vi "Camera.vi"(0 "Camera in":refnum<class "Camera.lvclass">, 1 "Stop":bool, 3 "Cluster":T1={"Bayer"={"Algorithm"=0, "Gain R"=1.0, "Gain B"=1.0, "Gain G"=1.0, "Pattern"=5}, "Acquisition Control"={"Trigger Selector"=0, "Acquisition Frame Rate"=0.0, "Exposure Time"=0.0, "Acquisition Frame Rate Target"=0.0}, "Analog Control"={"Black Level"=1.5, "Gain Selector"=10, "Gain"=1.0}} {"Analog Control"."Gain" min=1.0 max=15.0; "Analog Control"."Gain Selector" items=["Analog All"=10, "Digital All"=20]; "Analog Control"."Black Level" min=0.0 max=255.9375; "Acquisition Control"."Acquisition Frame Rate Target" min=0.001 max=150000000.0; "Acquisition Control"."Exposure Time" min=27.793333333333333 max=1048539.7933333333; "Acquisition Control"."Acquisition Frame Rate" min=0.9536888685435264 max=30.757874015748033; "Acquisition Control"."Trigger Selector" items=["Frame Start"=3, "Exposure Start"=10]; "Bayer"."Pattern" items=["Use hardware value"=5, "None"=0, "GB"=1, "GR"=2, "BG"=3, "RG"=4]; "Bayer"."Gain G" min=0.0 max=3.999; "Bayer"."Gain B" min=0.0 max=3.999; "Bayer"."Gain R" min=0.0 max=3.999; "Bayer"."Algorithm" items=["Bilinear", "VNG"]}, 4 "BCG Image Processing":T6={"Brightness"=128.0, "Contrast"=45.0, "Gamma"=1.0} {"Brightness" scale=0.0..400.0; "Contrast" scale=0.0..90.0; "Gamma" scale=0.005..5.0}, 5 "error in (no error)":errorcluster, 6 "Machine Vision":T7, 7 "Camera settings":T5={"Gamma"=1.0, "Gain"=7, "Sharpness"=0, "Contrast"=0.009999999999999995, "Exposure"=0.0004073180282999787} {"Exposure" min=0.000244140625 max=0.5 scale=0.0002..0.5; "Contrast" min=0.0 max=1.0 scale=0.001..1.0; "Sharpness" min=0 max=2 step=1 scale=0.0..2.0; "Gain" min=0 max=100 step=1 scale=0.1..100.0; "Gamma" min=0.01 max=10.0 scale=0.01..10.0}, 12 "Loop 0":bool, 13 "Override presets":bool) -> (9 "All Matches XY":sgl[][](array[numeric]), 11 "Used Edges (Adv. Straight Edge 1)":cluster{"Edge Information":T2[]}[](array[cluster]) {"Edge Information"."Distance (Real-World)" format="%.2f"; "Edge Information"."Location (Real-World)"."Y" format="%.2g"; "Edge Information"."Location (Real-World)"."X" format="%.2f"; "Edge Information"."Noise" format="%.2f"; "Edge Information"."Location (Pixel)"."Y" format="%.2g"; "Edge Information"."Location (Pixel)"."X" format="%.2f"; "Edge Information"."Strength" format="%.2f"; "Edge Information"."Distance (Pixel)" format="%.2f"}, 14 "Camera out":refnum<class "Camera.lvclass">, 15 "output cluster":T4, 16 "pattern matching":T3 {"Correlation Score" format="%.2f"; "Target Template Curve Score" format="%.2f"; "Template Target Curve Score" format="%.2f"; "Bounding Box"."y" format="%.2f"; "Bounding Box"."x" format="%.2f"; "Position"."y" format="%.2f"; "Position"."x" format="%.2f"; "Score" format="%.2f"; "Scale" format="%.2f"; "Angle" format="%.2f"; "Occlusion %" format="%.2f"}, 17 "Image":T8(plugin-control), 18 "Camera":dbl[](array[numeric]), 19 "error out":errorcluster)   [LabVIEW 2021, in "Camera.lvclass"]
uses:
  Camera.lvclass
  Machine Vision.ctl
  Image processing.ctl
  Camera settings.ctl
  <vilib>/vision/Pattern Matching.llb/IMAQ GM Match Report.ctl
  <vilib>/vision/Measure.llb/Edge New.ctl
  <vilib>/Analysis/baseanly.llb/Mean (DBL).vi
  <vilib>/Utility/file.llb/Read Delimited Spreadsheet (string).vi
  <vilib>/vision/NI_Vision_Development_Module.lvlib
  <vilib>/Analysis/NI_AALBase.lvlib
  <vilib>/vision/Pattern Matching.llb/IMAQ Match Range Setting.ctl
  <vilib>/vision/Shape Detection.llb/ShapeDetectionMatchOptions.ctl
  <vilib>/vision/Pattern Matching.llb/IMAQ Curve Parameters.ctl
panel:
  in  "Image Indicators":T4 {"Global Report"."Mean Value" format="%.2f"; "Global Report"."%" format="%.2f"; "Global Report"."Area (calibrated)" format="%.2f"; "Global Report"."Maximal Value" format="%.2f"; "Global Report"."Minimal Value" format="%.2f"; "Global Report"."Standard Variation" format="%.2f"}
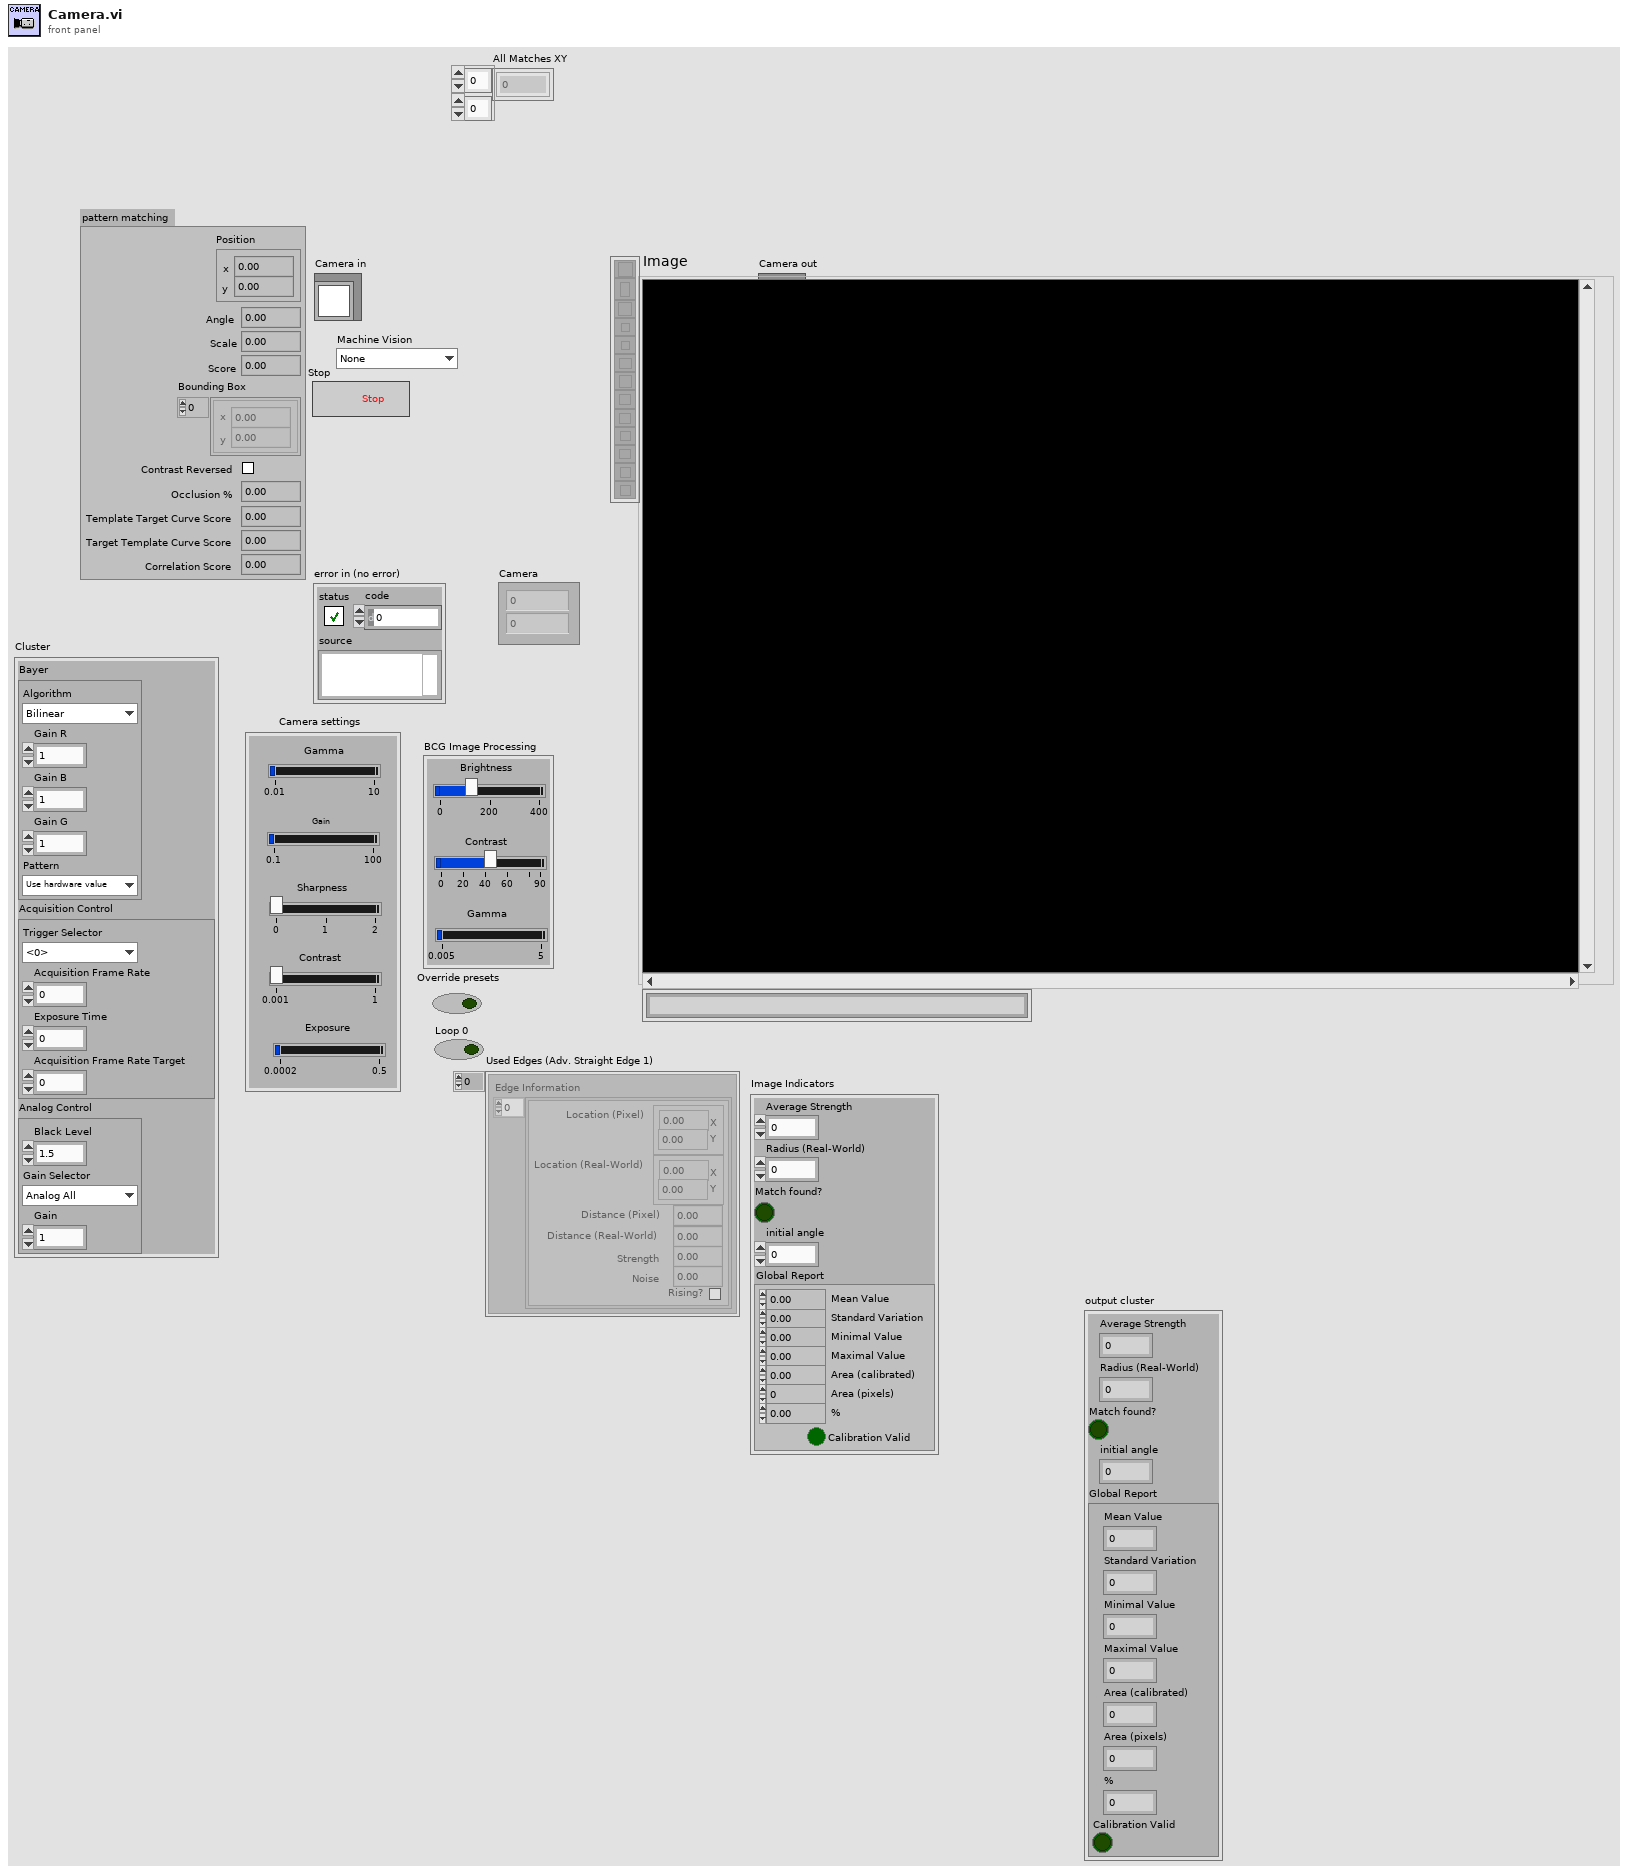
[diagram p1: front panel]
types:
  T1 = cluster{"Bayer":cluster{"Algorithm":u32, "Gain R":dbl, "Gain B":dbl, "Gain G":dbl, "Pattern":u32}, "Acquisition Control":cluster{"Trigger Selector":u32, "Acquisition Frame Rate":dbl, "Exposure Time":dbl, "Acquisition Frame Rate Target":dbl}, "Analog Control":cluster{"Black Level":dbl, "Gain Selector":u32, "Gain":dbl}}
  T2 = typedef "Edge New.ctl" = cluster{"Location (Pixel)":cluster{"X":sgl, "Y":sgl}, "Location (Real-World)":cluster{"X":sgl, "Y":sgl}, "Distance (Pixel)":dbl, "Distance (Real-World)":dbl, "Strength":dbl, "Noise":dbl, "Rising?":bool}
  T3 = typedef "IMAQ GM Match Report.ctl" = cluster{"Position":cluster{"x":sgl, "y":sgl}, "Angle":sgl, "Scale":sgl, "Score":sgl, "Bounding Box":cluster{"x":sgl, "y":sgl}[], "Contrast Reversed":bool, "Occlusion %":sgl, "Template Target Curve Score":sgl, "Target Template Curve Score":sgl, "Correlation Score":sgl}
  T4 = cluster{"Average Strength":dbl, "Radius (Real-World)":dbl, "Match found?":bool, "initial angle":sgl, "Global Report":cluster{"Mean Value":sgl, "Standard Variation":sgl, "Minimal Value":sgl, "Maximal Value":sgl, "Area (calibrated)":sgl, "Area (pixels)":u32, "%":sgl, "Calibration Valid":bool}}
  T5 = typedef "Camera.lvclass/Camera settings.ctl" = cluster{"Gamma":dbl, "Gain":i64, "Sharpness":i64, "Contrast":dbl, "Exposure":dbl}
  T6 = typedef "Camera.lvclass/Image processing.ctl" = cluster{"Brightness":sgl, "Contrast":sgl, "Gamma":sgl}
  T7 = typedef "Camera.lvclass/Machine Vision.ctl" = enum16{"None", "Assembly Tray Circle", "Assembly Tray Fiducial", "Partial Hexaboard", "sensor edge init", "HB edge init", "sensor edge pos1", "sensor edge pos2", "HB edge pos1", "HB edge pos2", "Sensor CH1-2", "HB CH1", "HB CH2", "V3 Sensor Circle", "Hexaboard Circle", "sensor CH1 check", "HB CH1 check ", "sensor ID"}
  T8 = typedef "IMAQ Image.ctl" = refnum<image>
  T9 = typedef "File Paths.ctl" = cluster{"Glue Pattern Folder":path, "Carrier Tray Folder":path, "Pick Up Tool Fixture Folder":path, "Components Folder":path, "Bellows Tool Offset.txt":path, "Pick Up Tool Offset.txt":path, "Dispense Tip Offset.txt":path, "Log Files":path, "Gantry Assembly Map.txt":path, "Syringe and offset map.txt":path, "Controllers Folder":path, "Local dbase config":path}
  T10 = typedef "IMAQ Curve Parameters.ctl" = cluster{"Extraction Mode":u32, "Edge Threshold":i32, "Edge Filter Size":u32, "Min Length":i32, "Row Search Step Size":i32, "Col Search Step Size":i32, "Max Endpoint Gap":i32, "Closed":bool, "Subpixel":bool}
  T11 = typedef "ShapeDetectionMatchOptions.ctl" = cluster{"Rotation":bool, "Scale":bool, "Occlusion":bool, "Range Settings":T12[]}
  T12 = typedef "IMAQ Match Range Setting.ctl" = cluster{"Match Constraints":u32, "Min":dbl, "Max":dbl}
  T13 = typedef "Image Type" = u32
  T14 = cluster{"Center (Pixels)":cluster{"X":sgl, "Y":sgl}, "Radius (Pixels)":dbl, "Center (Real-World)":cluster{"X":sgl, "Y":sgl}, "Radius (Real-World)":dbl, "Roundness (Real-World)":dbl, "Average Strength":dbl, "Average SNR (dB)":dbl}
  T15 = cluster{"Position":cluster{"X":sgl, "Y":sgl}, "Radius":dbl, "Score":dbl}[]
  T16 = cluster{"Position":cluster{"X":sgl, "Y":sgl}, "Radius":dbl, "Score":dbl}
  T17 = cluster{"Pos. X":i32, "Pos. Y":i32, "Radius":i32, "Core Area":i32}[]
  T18 = cluster{"Pos. X":i32, "Pos. Y":i32, "Radius":i32, "Core Area":i32}
  T19 = cluster{"Position":cluster{"x":sgl, "y":sgl}, "Angle":sgl, "Scale":sgl, "Score":sgl, "Bounding Box":cluster{"x":sgl, "y":sgl}[]}[]
  T20 = cluster{"Position":cluster{"x":sgl, "y":sgl}, "Angle":sgl, "Scale":sgl, "Score":sgl, "Bounding Box":cluster{"x":sgl, "y":sgl}[]}
  T21 = cluster{"Mean Value":sgl, "Standard Variation":sgl, "Minimal Value":sgl, "Maximal Value":sgl, "Area (calibrated)":sgl, "Area (pixels)":u32, "%":sgl, "Calibration Valid":bool}
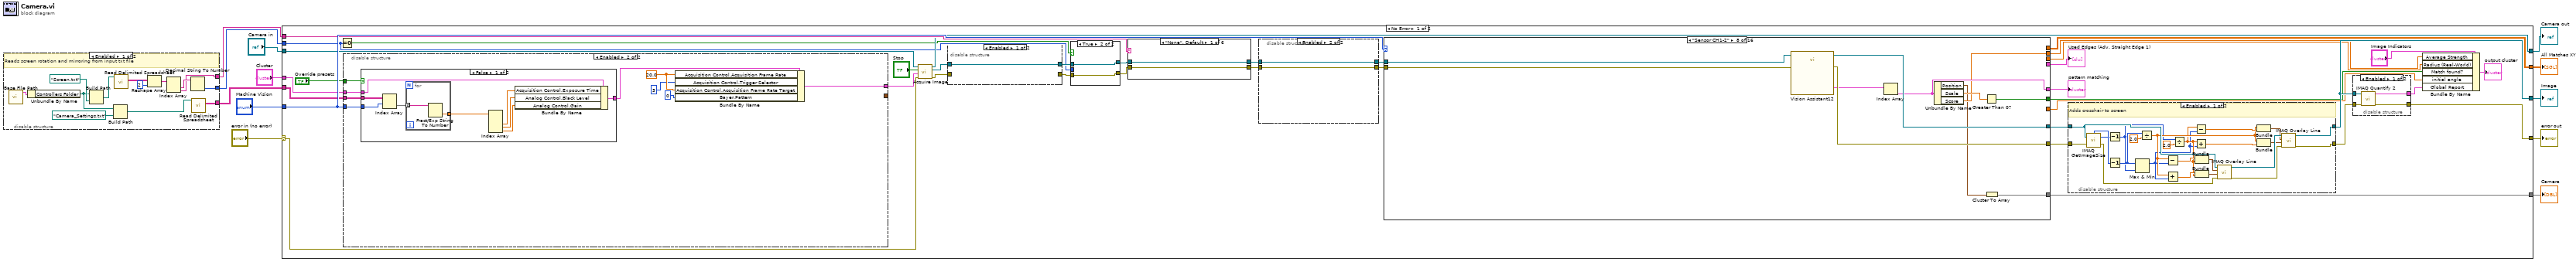
[diagram p0: block diagram]
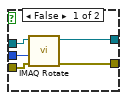
[diagram p3: hidden frame]
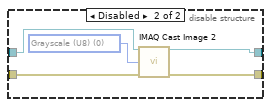
[diagram p4: hidden frame]
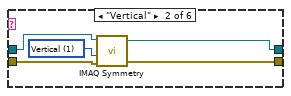
[diagram p5: hidden frame]
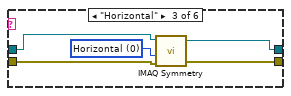
[diagram p6: hidden frame]
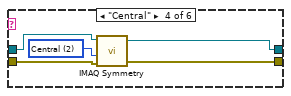
[diagram p7: hidden frame]
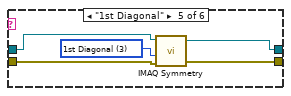
[diagram p8: hidden frame]
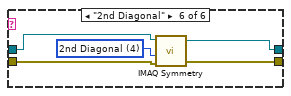
[diagram p9: hidden frame]
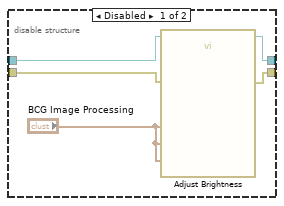
[diagram p12: hidden frame]
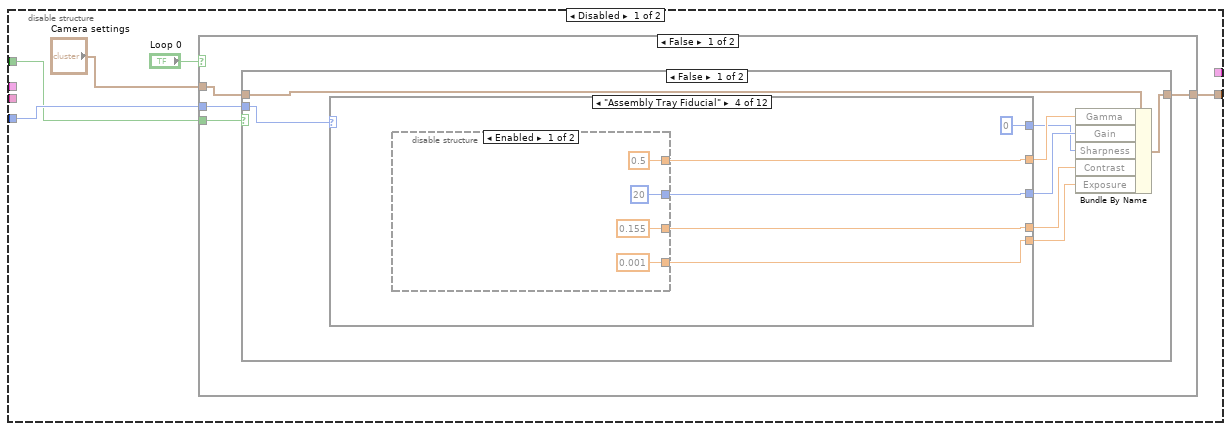
[diagram p13: hidden frame]
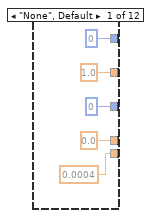
[diagram p14: hidden frame]
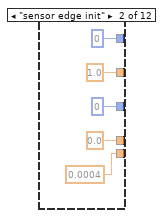
[diagram p15: hidden frame]
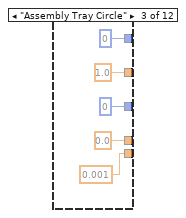
[diagram p16: hidden frame]
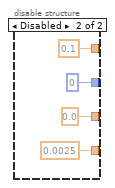
[diagram p17: hidden frame]
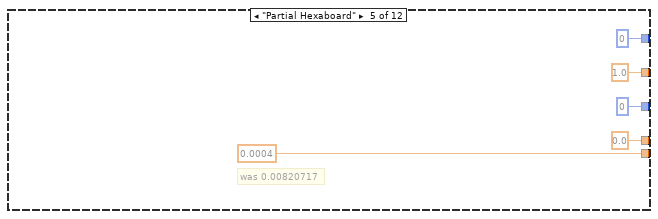
[diagram p18: hidden frame]
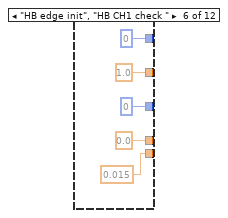
[diagram p19: hidden frame]
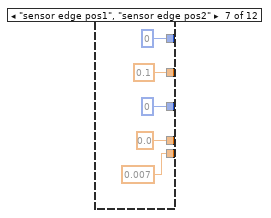
[diagram p20: hidden frame]
diagram:
  n1 = disable-structure shown="Enabled" {
    disable-tunnel: [w18 _] -> w6
    disable-tunnel: [w17 _] -> w5
    disable-tunnel: [w13 _] -> w2
    frame Enabled {
      # "Reads screen rotation and mirroring from input txt file"
      n2 = call "Base File Path.vi"() -> ("Paths Out"=w25:T9)  [unwired: 11 in]
      n3 = Unbundle By Name(w25) -> ("Controllers Folder"=w15:path)
      n4 = Build Path(base path=w15, name or relative path=path "Screen.txt") -> (appended path=w23:path)
      n5 = Build Path(base path=w15, name or relative path=path "Camera_Settings.txt") -> (appended path=w14:path)
      n6 = call-poly <vilib>:"Read Delimited Spreadsheet.vi"("file path (dialog if empty)"=w23) -> ("all rows"=w22:string[][])  [unwired: 9 in, 5 out]
      n7 = Reshape Array(w22, 2 ("dimension size")) -> (w20:string[])
      n8 = Index Array(array=w20) -> (element #1=w19:string, element #2=w17:string)  [unwired: 2 in]
      n9 = Decimal String To Number(string=w19) -> (number=w18:i32)  [unwired: 2 in, 1 out]
      n10 = call-poly <vilib>:"Read Delimited Spreadsheet.vi"("file path (dialog if empty)"=w14) -> ("all rows"=w13:string[][])  [unwired: 9 in, 5 out]
    }
    frame Disabled {
    }
  }
  n11 = case shown="No Error" "error in (no error)" {
    selector: "error in (no error)" -> [w46 w627]
    tunnel: [w51 w627] -> w11
    tunnel: [w48 w626] -> w10
    tunnel: "Camera in" -> [w49 w626]
    tunnel: [w63 _] -> w4
    tunnel: [w58 _] -> w8
    tunnel: "Machine Vision" -> [w62 _]
    tunnel: w6 -> [w32 _]
    tunnel: w5 -> [w50 _]
    tunnel: "Cluster" -> [w29 _]
    tunnel: w2 -> [w27 _]
    tunnel: [w26 _] -> w1
    frame No Error {
      n12 = Equal To 0?(x=w32) -> (x = 0?=w31:bool)
      n13 = disable-structure shown="Enabled" {
        disable-tunnel: w62 -> [w146 w241]
        disable-tunnel: [w145 _] -> _
        disable-tunnel: "Override presets" -> [w142 w243]
        disable-tunnel: w29 -> [_ w242]
        disable-tunnel: [_ w238] -> w28
        disable-tunnel: w27 -> [_ w240]
        frame Disabled {
          n14 = case shown="False" "Loop 0" {
            tunnel: w142 -> [w150 _]
            tunnel: w146 -> [w149 _]
            tunnel: "Camera settings" -> [w148 w234]
            tunnel: [w147 w233] -> w145
            frame False {
              n15 = case shown="False" w150 {
                tunnel: w149 -> [w158 _]
                tunnel: w148 -> [w157 w227]
                tunnel: [w151 w227] -> w147
                frame False {
                  n16 = case shown="\"Assembly Tray Fiducial\"" w158 {
                    tunnel: [1.0 ("Gamma::Value") 1.0 ("Gamma::Value") 1.0 ("Gamma::Value") w178 1.0 ("Gamma::Value") 1.0 ("Gamma::Value") 0.1 ("Gamma::Value") 0.6 ("Gamma::Value") 1.0 ("Gamma::Value") 0.1 ("Gamma::Value") 0.25 ("Gamma::Value") 0.01 ("Gamma::Value")] -> w156
                    tunnel: [i64 0 ("Gain::Value") i64 0 ("Gain::Value") i64 0 ("Gain::Value") w177 i64 0 ("Gain::Value") i64 0 ("Gain::Value") i64 0 ("Gain::Value") i64 0 ("Gain::Value") i64 0 ("Gain::Value") i64 0 ("Gain::Value") i64 0 ("Gain::Value") i64 0 ("Gain::Value")] -> w155
                    tunnel: [i64 0 ("Sharpness::Value") i64 0 ("Sharpness::Value") i64 0 ("Sharpness::Value") i64 0 ("Sharpness::Value") i64 0 ("Sharpness::Value") i64 0 ("Sharpness::Value") i64 0 ("Sharpness::Value") i64 0 ("Sharpness::Value") i64 0 ("Sharpness::Value") i64 0 ("Sharpness::Value") i64 0 ("Sharpness::Value") i64 0 ("Sharpness::Value")] -> w154
                    tunnel: [0.0 ("Contrast::Value") 0.0 ("Contrast::Value") 0.0 ("Contrast::Value") w175 0.0 ("Contrast::Value") 0.0 ("Contrast::Value") 0.0 ("Contrast::Value") 0.0 ("Contrast::Value") 0.0 ("Contrast::Value") 0.0 ("Contrast::Value") 0.0 ("Contrast::Value") 0.0 ("Contrast::Value")] -> w153
                    tunnel: [0.0004 ("Exposure::Value") 0.0004 ("Exposure::Value") 0.001 ("Exposure::Value") w174 0.0004 ("Exposure::Value") 0.015 ("Exposure::Value") 0.007 ("Exposure::Value") 0.015 ("Exposure::Value") 0.001 ("Exposure::Value") 0.025 ("Exposure::Value") 0.03 ("Exposure::Value") 0.03 ("Exposure::Value")] -> w152
                    frame "None", Default {
                    }
                    frame "sensor edge init" {
                    }
                    frame "Assembly Tray Circle" {
                    }
                    frame "Assembly Tray Fiducial" {
                      n17 = disable-structure shown="Enabled" {
                        disable-tunnel: [0.5 ("Gamma::Value") 0.1 ("Gamma::Value")] -> w178
                        disable-tunnel: [i64 20 ("Gain::Value") i64 0 ("Gain::Value")] -> w177
                        disable-tunnel: [0.155 ("Contrast::Value") 0.0 ("Contrast::Value")] -> w175
                        disable-tunnel: [0.001 ("Exposure::Value") 0.0025 ("Exposure::Value")] -> w174
                        frame Enabled {
                        }
                        frame Disabled {
                        }
                      }
                    }
                    frame "Partial Hexaboard" {
                      # "was 0.00820717"
                    }
                    frame "HB edge init", "HB CH1 check " {
                    }
                    frame "sensor edge pos1", "sensor edge pos2" {
                    }
                    frame "HB edge pos1", "HB edge pos2" {
                    }
                    frame "Sensor CH1-2", "V3 Sensor Circle", "sensor CH1 check" {
                    }
                    frame "HB CH1" {
                    }
                    frame "Hexaboard Circle" {
                    }
                    frame "HB CH2" {
                    }
                  }
                  n18 = Bundle By Name(cluster=w157, "Gamma"=w156, "Gain"=w155, "Sharpness"=w154, "Contrast"=w153, "Exposure"=w152) -> (w151:T5)
                }
                frame True {
                }
              }
            }
            frame True {
              n19 = Bundle By Name(cluster=w234, "Gamma"=1.0, "Gain"=i64 0, "Sharpness"=i64 0, "Contrast"=0.0, "Exposure"=0.0004) -> (w233:T5)
            }
          }
        }
        frame Enabled {
          w237 = 20.0 ("Acquisition Control.Acquisition Frame Rate Target")
          n20 = case shown="False" w243 {
            tunnel: w242 -> [w251 w255]
            tunnel: [w252 w255] -> w239
            tunnel: w241 -> [w246 _]
            tunnel: w240 -> [w250 _]
            frame False {
              n21 = Index Array(array=w250, index (row)=w246) -> (element=w245:string[])  [unwired: 1 in]
              n22 = for {
                tunnel: w245 -> [w254] mode=indexing
                tunnel: [w253] -> w244 mode=indexing
                n23 = Fract/Exp String To Number(string=w254) -> (number=w253:dbl)  [unwired: 3 in, 1 out]
              }
              n24 = Index Array(array=w244) -> (element #2=w249:dbl, element #3=w248:dbl, element #4=w247:dbl)  [unwired: 4 in, 1 out]
              n25 = Bundle By Name(cluster=w251, "Acquisition Control.Exposure Time"=w249, "Analog Control.Black Level"=w248, "Analog Control.Gain"=w247) -> (w252:T1)
            }
            frame True {
            }
          }
          n26 = Bundle By Name(cluster=w239, "Acquisition Control.Acquisition Frame Rate"=w237, "Acquisition Control.Trigger Selector"=u32 3, "Acquisition Control.Acquisition Frame Rate Target"=w237, "Bayer.Pattern"=u32 0) -> (w238:T1)
        }
      }
      n27 = call-dynamic "Acquire Image.vi"("error in (no error)"=w46, "Cluster"=w28, "Stop"="Stop", "Camera in"=w49) -> ("error out"=w37:errorcluster, "Image Out"=w39:T8, "Camera out"=w48:refnum<class "Camera.lvclass">)  [unwired: 5 in]
      n28 = disable-structure shown="Enabled" {
        disable-tunnel: w39 -> [w71 w75]
        disable-tunnel: [w71 w74] -> w38
        disable-tunnel: w37 -> [_ w73]
        disable-tunnel: [_ w72] -> w36
        frame Enabled {
        }
        frame Disabled {
          w76 = T13 0 items=["Grayscale (U8)", "Grayscale (I16)", "Grayscale (SGL)", "Complex (CSG)", "RGB (U32)", "HSL (U32)", "RGB (U64)", "Grayscale (U16)"] ("Image Type")
          n29 = call "IMAQ Cast Image 2"("Image Src"=w75, "Image Type"=w76, "error in (no error)"=w73) -> ("Image Dst Out"=w74:T8, "error out"=w72:errorcluster)  [unwired: 11 in]
        }
      }
      n30 = case shown="True" w31 {
        tunnel: [w68 w69] -> w54
        tunnel: [w67 w70] -> w53
        tunnel: w38 -> [w66 w70]
        tunnel: w36 -> [w65 w69]
        tunnel: w32 -> [w64 _]
        frame False {
          n31 = call "IMAQ Rotate"("error in (no error)"=w65, "Angle (degrees)"=w64, "Image Src"=w66) -> ("error out"=w68:errorcluster, "Image Dst Out"=w67:T8)  [unwired: 7 in]
        }
        frame True {
        }
      }
      n32 = case shown="\"None\", Default" w50 {
        tunnel: [w78 w83 w88 w93 w98 w103] -> w61
        tunnel: [w77 w82 w87 w92 w97 w102] -> w57
        tunnel: w54 -> [w77 w81 w86 w91 w96 w101]
        tunnel: w53 -> [w78 w80 w85 w90 w95 w100]
        frame "None", Default {
        }
        frame "Vertical" {
          w79 = u32 1 items=["Horizontal", "Vertical", "Central", "1st Diagonal", "2nd Diagonal"] ("Type of Symmetry")
          n33 = call "IMAQ Symmetry"("error in (no error)"=w81, "Type of Symmetry"=w79, "Image Src"=w80) -> ("error out"=w82:errorcluster, "Image Dst Out"=w83:T8)  [unwired: 2 in]
        }
        frame "Horizontal" {
          w84 = u32 0 items=["Horizontal", "Vertical", "Central", "1st Diagonal", "2nd Diagonal"] ("Type of Symmetry")
          n34 = call "IMAQ Symmetry"("error in (no error)"=w86, "Type of Symmetry"=w84, "Image Src"=w85) -> ("error out"=w87:errorcluster, "Image Dst Out"=w88:T8)  [unwired: 2 in]
        }
        frame "Central" {
          w89 = u32 2 items=["Horizontal", "Vertical", "Central", "1st Diagonal", "2nd Diagonal"] ("Type of Symmetry")
          n35 = call "IMAQ Symmetry"("error in (no error)"=w91, "Type of Symmetry"=w89, "Image Src"=w90) -> ("error out"=w92:errorcluster, "Image Dst Out"=w93:T8)  [unwired: 2 in]
        }
        frame "1st Diagonal" {
          w94 = u32 3 items=["Horizontal", "Vertical", "Central", "1st Diagonal", "2nd Diagonal"] ("Type of Symmetry")
          n36 = call "IMAQ Symmetry"("error in (no error)"=w96, "Type of Symmetry"=w94, "Image Src"=w95) -> ("error out"=w97:errorcluster, "Image Dst Out"=w98:T8)  [unwired: 2 in]
        }
        frame "2nd Diagonal" {
          w99 = u32 4 items=["Horizontal", "Vertical", "Central", "1st Diagonal", "2nd Diagonal"] ("Type of Symmetry")
          n37 = call "IMAQ Symmetry"("error in (no error)"=w101, "Type of Symmetry"=w99, "Image Src"=w100) -> ("error out"=w102:errorcluster, "Image Dst Out"=w103:T8)  [unwired: 2 in]
        }
      }
      n38 = disable-structure shown="Enabled" {
        disable-tunnel: w61 -> [w139 w140]
        disable-tunnel: [w137 w140] -> w60
        disable-tunnel: w57 -> [w136 w141]
        disable-tunnel: [w135 w141] -> w56
        frame Disabled {
          n39 = call "Adjust Brightness"("Image In"=w139, "Red BCG Values (Brightness 1)"="BCG Image Processing", "Green BCG Values (Brightness 1)"="BCG Image Processing", "Blue BCG Values (Brightness 1)"="BCG Image Processing", "error in"=w136) -> ("Image Out"=w137:T8, "error out"=w135:errorcluster)  [unwired: 21 in]
        }
        frame Enabled {
        }
      }
      n40 = case shown="\"Sensor CH1-2\"" w62 {
        tunnel: [w256 w262 w278 w291 w314 w337 w360 w381 w396 w463 w482 w524 w560 w574 w588 w607] -> w63
        tunnel: [w261 w273 w284 w304 w327 w350 w373 w391 w400 w464 w490 w531 w572 w586 w594 w613] -> w59
        tunnel: w60 -> [w261 w274 w283 w305 w328 w351 w374 w390 w399 w467 w489 w530 w571 w585 w593 w612]
        tunnel: [0.0 ("Radius (Real-World)") w264 w281 _ _ _ _ _ w392 _ w484 w526 w568 w577 _ _] -> w43
        tunnel: [0.0 ("Strength") w271 w282 w297 w318 w341 w364 w383 w393 _ w483 w525 w570 w584 _ _] -> w44
        tunnel: w56 -> [w260 w270 w279 w306 w329 w352 w375 w388 w397 w465 w487 w528 w569 w582 w591 w610]
        tunnel: [w260 w269 w280 w295 w320 w342 w366 w389 w398 w466 w488 w529 w562 w583 w592 w611] -> w55
        tunnel: [_ w265 _ w289 w312 w335 w358 w384 w394 _ w485 w527 w563 w576 w589 w608] -> w42
        tunnel: [_ _ _ w302 w325 w348 w371 _ _ _ _ _ _ _ _ _] -> w41
        tunnel: [_ _ _ _ _ _ _ w386 w395 _ w486 _ _ _ w590 w609] -> w34
        tunnel: [_ _ _ _ _ w344 _ _ _ _ _ _ _ _ _ _] -> w33
        tunnel: [_ _ _ _ _ _ _ _ _ w462 _ _ _ _ _ _] -> w26
        frame "None", "sensor edge init", "HB edge init", Default {
          n41 = Initialize Array(0.0 ("element")) -> (w256:dbl[])  [unwired: 1 in]
        }
        frame "Assembly Tray Circle" {
          n42 = call "Vision Assistant"("Image In"=w274, "error in"=w270) -> ("Image Out"=w273:T8, "Fitted Circle (Find Circular Edge 1)"=w272:T14, "error out"=w269:errorcluster)  [unwired: 23 in]
          n43 = Unbundle By Name(w272) -> ("Center (Real-World)"=w275:cluster{"X":sgl, "Y":sgl}, "Average Strength"=w271:dbl, "Radius (Real-World)"=w264:dbl)
          n44 = Greater?(x=w264, y=0.046) -> (0:w263:bool)
          n45 = Less?(x=w264, y=0.048) -> (x < y?=w266:bool)
          n46 = Unbundle By Name(w275) -> ("X"=w277:sgl, "Y"=w276:sgl)
          n47 = And(x=w263, y=w266) -> (x .and. y?=w265:bool)
          n48 = Build Array(w277, w276) -> (w262:sgl[])
        }
        frame "Partial Hexaboard" {
          n49 = call "Vision Assistant20"("Image In"=w283, "error in"=w279) -> ("Image Out"=w284:T8, "Fitted Circle (Find Circular Edge 1)"=w286:T14, "error out"=w280:errorcluster)  [unwired: 23 in]
          n50 = Unbundle By Name(w286) -> ("Center (Real-World)"=w288:cluster{"X":sgl, "Y":sgl}, "Average Strength"=w282:dbl, "Radius (Real-World)"=w281:dbl)
          n51 = Unbundle By Name(w288) -> ("X"=w287:sgl, "Y"=w285:sgl)
          n52 = Build Array(w287, w285) -> (w278:sgl[])
        }
        frame "sensor edge pos1" {
          w300 = 0 ("index (row)")
          n53 = call "Vision Assistant6"("Image In"=w305, "error in"=w306) -> ("Image Out"=w304:T8, "Calibrated Results (Caliper 1)"=w303:sgl[][], "Calibrated Results (Caliper 2)"=w301:sgl[][], "Used Edges (Adv. Straight Edge 1)"=w298:cluster{"Edge Information":T2[]}[], "error out"=w296:errorcluster)  [unwired: 19 in, 2 out]
          n54 = Index Array(array=w298) -> (element=w294:cluster{"Edge Information":T2[]})  [unwired: 1 in]
          n55 = Index Array(array=w303, index (row)=w300, index (col)=w300) -> (element=w302:sgl)
          n56 = Index Array(array=w301, index (row)=0 ("disabled index (col)")) -> (element=w291:sgl[])  [unwired: 1 in]
          n57 = Unbundle By Name(w294) -> ("Edge Information"=w293:T2[])
          n58 = for {
            tunnel: w293 -> [w311] mode=indexing
            tunnel: [w310] -> w292 mode=indexing
            n59 = Unbundle By Name(w311) -> ("Strength"=w310:dbl)
          }
          n60 = call <vilib>:"Clear Errors.vi"("error in (no error)"=w296) -> ("error out"=w295:errorcluster)  [unwired: 5 in, 1 out]
          n61 = Empty Array?(array=w292) -> (empty?=w290:bool)
          n62 = case shown="False" w290 {
            tunnel: w292 -> [w308 _]
            tunnel: [w307 0.0 ("mean")] -> w297
            frame False {
              n63 = call-poly <vilib>:"Mean.vi"("X"=w308) -> ("mean"=w307:dbl)  [unwired: 1 out]
            }
            frame True {
            }
          }
          n64 = Not(x=w290) -> (.not. x?=w289:bool)
        }
        frame "sensor edge pos2" {
          w323 = 0 ("index (row)")
          n65 = call "Vision Assistant8"("Image In"=w328, "error in"=w329) -> ("Image Out"=w327:T8, "Calibrated Results (Caliper 1)"=w326:sgl[][], "Calibrated Results (Caliper 2)"=w324:sgl[][], "Used Edges (Adv. Straight Edge 1)"=w319:cluster{"Edge Information":T2[]}[], "error out"=w321:errorcluster)  [unwired: 21 in]
          n66 = Index Array(array=w319) -> (element=w317:cluster{"Edge Information":T2[]})  [unwired: 1 in]
          n67 = Index Array(array=w326, index (row)=w323, index (col)=w323) -> (element=w325:sgl)
          n68 = Index Array(array=w324, index (row)=0 ("disabled index (col)")) -> (element=w314:sgl[])  [unwired: 1 in]
          n69 = Unbundle By Name(w317) -> ("Edge Information"=w316:T2[])
          n70 = for {
            tunnel: w316 -> [w334] mode=indexing
            tunnel: [w333] -> w315 mode=indexing
            n71 = Unbundle By Name(w334) -> ("Strength"=w333:dbl)
          }
          n72 = call <vilib>:"Clear Errors.vi"("error in (no error)"=w321) -> ("error out"=w320:errorcluster)  [unwired: 5 in, 1 out]
          n73 = Empty Array?(array=w315) -> (empty?=w313:bool)
          n74 = case shown="True" w313 {
            tunnel: w315 -> [w331 _]
            tunnel: [w330 0.0 ("mean")] -> w318
            frame False {
              n75 = call-poly <vilib>:"Mean.vi"("X"=w331) -> ("mean"=w330:dbl)  [unwired: 1 out]
            }
            frame True {
            }
          }
          n76 = Not(x=w313) -> (.not. x?=w312:bool)
        }
        frame "HB edge pos1" {
          w346 = 0 ("index (row)")
          n77 = call "Vision Assistant5"("Image In"=w351, "error in"=w352) -> ("Image Out"=w350:T8, "Calibrated Results (Caliper 1)"=w349:sgl[][], "Calibrated Results (Caliper 2)"=w347:sgl[][], "Used Edges (Adv. Straight Edge 1)"=w344:cluster{"Edge Information":T2[]}[], "error out"=w343:errorcluster)  [unwired: 21 in]
          n78 = Index Array(array=w344) -> (element=w340:cluster{"Edge Information":T2[]})  [unwired: 1 in]
          n79 = Index Array(array=w349, index (row)=w346, index (col)=w346) -> (element=w348:sgl)
          n80 = Index Array(array=w347, index (row)=0 ("disabled index (col)")) -> (element=w337:sgl[])  [unwired: 1 in]
          n81 = Unbundle By Name(w340) -> ("Edge Information"=w339:T2[])
          n82 = for {
            tunnel: w339 -> [w357] mode=indexing
            tunnel: [w356] -> w338 mode=indexing
            n83 = Unbundle By Name(w357) -> ("Strength"=w356:dbl)
          }
          n84 = call <vilib>:"Clear Errors.vi"("error in (no error)"=w343) -> ("error out"=w342:errorcluster)  [unwired: 5 in, 1 out]
          n85 = Empty Array?(array=w338) -> (empty?=w336:bool)
          n86 = case shown="True" w336 {
            tunnel: w338 -> [w354 _]
            tunnel: [w353 0.0 ("mean")] -> w341
            frame False {
              n87 = call-poly <vilib>:"Mean.vi"("X"=w354) -> ("mean"=w353:dbl)  [unwired: 1 out]
            }
            frame True {
            }
          }
          n88 = Not(x=w336) -> (.not. x?=w335:bool)
        }
        frame "HB edge pos2" {
          w369 = 0 ("index (row)")
          n89 = call "Vision Assistant10"("Image In"=w374, "error in"=w375) -> ("Image Out"=w373:T8, "Calibrated Results (Caliper 1)"=w372:sgl[][], "Calibrated Results (Caliper 2)"=w370:sgl[][], "Used Edges (Adv. Straight Edge 1)"=w365:cluster{"Edge Information":T2[]}[], "error out"=w367:errorcluster)  [unwired: 21 in]
          n90 = Index Array(array=w365) -> (element=w363:cluster{"Edge Information":T2[]})  [unwired: 1 in]
          n91 = Index Array(array=w372, index (row)=w369, index (col)=w369) -> (element=w371:sgl)
          n92 = Index Array(array=w370, index (row)=0 ("disabled index (col)")) -> (element=w360:sgl[])  [unwired: 1 in]
          n93 = Unbundle By Name(w363) -> ("Edge Information"=w362:T2[])
          n94 = for {
            tunnel: w362 -> [w380] mode=indexing
            tunnel: [w379] -> w361 mode=indexing
            n95 = Unbundle By Name(w380) -> ("Strength"=w379:dbl)
          }
          n96 = call <vilib>:"Clear Errors.vi"("error in (no error)"=w367) -> ("error out"=w366:errorcluster)  [unwired: 5 in, 1 out]
          n97 = Empty Array?(array=w361) -> (empty?=w359:bool)
          n98 = case shown="True" w359 {
            tunnel: w361 -> [w377 _]
            tunnel: [w376 0.0 ("mean")] -> w364
            frame False {
              n99 = call-poly <vilib>:"Mean.vi"("X"=w377) -> ("mean"=w376:dbl)  [unwired: 1 out]
            }
            frame True {
            }
          }
          n100 = Not(x=w359) -> (.not. x?=w358:bool)
        }
        frame "Sensor CH1-2" {
          n101 = call "Vision Assistant12"("Image In"=w390, "error in"=w388) -> ("Image Out"=w391:T8, "Calibrated Matches (Pattern Matching 1)"=w387:T3[], "error out"=w389:errorcluster)  [unwired: 22 in, 1 out]
          n102 = Index Array(array=w387) -> (element=w386:T3)  [unwired: 1 in]
          n103 = Unbundle By Name(w386) -> ("Position"=w382:cluster{"x":sgl, "y":sgl}, "Scale"=w385:sgl, "Score"=w383:sgl)
          n104 = Greater Than 0?(x=w385) -> (x > 0?=w384:bool)
          n105 = Cluster To Array(cluster=w382) -> (array=w381:sgl[])
        }
        frame "Assembly Tray Fiducial" {
          n106 = disable-structure shown="Enabled" {
            disable-tunnel: [w411 w419 w435] -> w400
            disable-tunnel: w399 -> [w410 w420 w436]
            disable-tunnel: [w409 w415 w438] -> w398
            disable-tunnel: w397 -> [w408 w429 w437]
            disable-tunnel: [w401 w417 w432] -> w396
            disable-tunnel: [w406 _ _] -> w395
            disable-tunnel: [w404 w427 w439] -> w394
            disable-tunnel: [w403 w414 w433] -> w393
            disable-tunnel: [_ w413 w431] -> w392
            frame Enabled {
              n107 = call "Vision Assistant13"("Image In"=w410, "error in"=w408) -> ("Image Out"=w411:T8, "Calibrated Matches (Pattern Matching 1)"=w407:T3[], "error out"=w409:errorcluster)  [unwired: 22 in, 1 out]
              n108 = Index Array(array=w407) -> (element=w406:T3)  [unwired: 1 in]
              n109 = Unbundle By Name(w406) -> ("Position"=w402:cluster{"x":sgl, "y":sgl}, "Scale"=w405:sgl, "Score"=w403:sgl)
              n110 = Cluster To Array(cluster=w402) -> (array=w401:sgl[])
              n111 = Greater Than 0?(x=w405) -> (x > 0?=w404:bool)
            }
            frame Disabled {
              n112 = call-poly "IMAQ Detect Shapes"("Curve Parameters"=T10 {"Extraction Mode"=0, "Edge Threshold"=30, "Edge Filter Size"=1, "Min Length"=25, "Row Search Step Size"=15, "Col Search Step Size"=15, "Max Endpoint Gap"=10, "Closed"=FALSE, "Subpixel"=FALSE}, "error in (no error)"=w429, "Match Options"=T11 {"Rotation"=FALSE, "Scale"=FALSE, "Occlusion"=TRUE, "Range Settings"=[{"Match Constraints"=2, "Min"=0.0, "Max"=25.0}]}, "Circle Descriptor"=cluster{"Min Radius":dbl, "Max Radius":dbl} {"Min Radius"=105.0, "Max Radius"=115.0}, "Image"=w420) -> ("error out"=w424:errorcluster, "Number of Matches Returned"=w428:i32, "Circles"=w423:T15)  [unwired: 4 in]
              n113 = Index Array(array=w423) -> (element=w422:T16)  [unwired: 1 in]
              n114 = Greater Than 0?(x=w428) -> (x > 0?=w427:bool)
              n115 = Unbundle By Name(w422) -> ("Position"=w421:cluster{"X":sgl, "Y":sgl}, "Radius"=w413:dbl, "Score"=w414:dbl)
              n116 = call "IMAQ Convert Pixel to Real World"("error in (no error)"=w424, "Pixel Coordinates"=w421, "Calibrated Image"=w420) -> ("error out"=w416:errorcluster, "Real World Coordinates"=w418:cluster{"X":sgl, "Y":sgl}, "Calibrated Image (duplicate)"=w419:T8)  [unwired: 3 in, 3 out]
              n117 = Cluster To Array(cluster=w418) -> (array=w417:sgl[])
              n118 = call <vilib>:"Clear Errors.vi"("error in (no error)"=w416) -> ("error out"=w415:errorcluster)  [unwired: 5 in, 1 out]
            }
            frame Disabled {
              n119 = call "Vision Assistant14"("Image In"=w436, "error in"=w437) -> ("Image Out"=w435:T8, "Circles Calibrated (Shape Detection 1)"=w434:T15, "Number of Matches (Shape Detection 1)"=w430:i32, "error out"=w438:errorcluster)  [unwired: 21 in, 1 out]
              n120 = case shown="1" w430 {
                tunnel: w434 -> [_ w448 w456]
                tunnel: [0.0 w444 w454] -> w433
                tunnel: [sgl[] [] ("Position") w445 w451] -> w432
                tunnel: [0.0 ("Radius") w443 w449] -> w431
                frame 0 {
                }
                frame 1 {
                  n121 = Index Array(array=w448) -> (element=w447:T16)  [unwired: 1 in]
                  n122 = Unbundle By Name(w447) -> ("Position"=w446:cluster{"X":sgl, "Y":sgl}, "Radius"=w443:dbl, "Score"=w444:dbl)
                  n123 = Cluster To Array(cluster=w446) -> (array=w445:sgl[])
                }
                frame 2, Default {
                  n124 = for {
                    tunnel: w456 -> [w461] mode=indexing
                    tunnel: [w459] -> w452 mode=indexing
                    tunnel: [w458] -> w450 mode=indexing
                    tunnel: [w457] -> w455 mode=indexing
                    n125 = Unbundle By Name(w461) -> ("Position"=w460:cluster{"X":sgl, "Y":sgl}, "Radius"=w458:dbl, "Score"=w457:dbl)
                    n126 = Cluster To Array(cluster=w460) -> (array=w459:sgl[])
                  }
                  n127 = Array Max & Min(array=w455) -> (max value=w454:dbl, max index (indices)=w453:i32)  [unwired: 2 out]
                  n128 = Index Array(array=w450, index=w453) -> (element=w449:dbl)
                  n129 = Index Array(array=w452, index (row)=w453) -> (element=w451:sgl[])  [unwired: 1 in]
                }
              }
              n130 = Greater Than 0?(x=w430) -> (x > 0?=w439:bool)
            }
          }
        }
        frame "sensor ID" {
          n131 = disable-structure shown="Enabled" {
            disable-tunnel: w467 -> [w474 w480]
            disable-tunnel: [w473 w481] -> w466
            disable-tunnel: w465 -> [w472 w481]
            disable-tunnel: [w471 w480] -> w464
            disable-tunnel: [w469 sgl[] [] ("Position")] -> w463
            disable-tunnel: [w468 sgl[][] [] ("Position")] -> w462
            frame Disabled {
              n132 = call "Vision Assistant15"("Image In"=w474, "error in"=w472) -> ("Image Out"=w471:T8, "Calibrated Matches (Pattern Matching 1)"=w470:T3[], "error out"=w473:errorcluster)  [unwired: 22 in, 1 out]
              n133 = for {
                tunnel: w470 -> [w477] mode=indexing
                tunnel: [w475] -> w468 mode=indexing
                n134 = Unbundle By Name(w477) -> ("Position"=w476:cluster{"x":sgl, "y":sgl})
                n135 = Cluster To Array(cluster=w476) -> (array=w475:sgl[])
              }
              n136 = Index Array(array=w468) -> (element=w469:sgl[])  [unwired: 2 in]
            }
            frame Enabled {
            }
          }
        }
        frame "HB CH1" {
          n137 = disable-structure shown="Enabled" {
            disable-tunnel: [w501 w502] -> w490
            disable-tunnel: w489 -> [w500 w504]
            disable-tunnel: [w499 w508] -> w488
            disable-tunnel: w487 -> [w498 w515]
            disable-tunnel: [w491 w520] -> w482
            disable-tunnel: [w496 _] -> w486
            disable-tunnel: [w494 w519] -> w485
            disable-tunnel: [_ w505] -> w484
            disable-tunnel: [w493 _] -> w483
            frame Enabled {
              n138 = call "Vision Assistant7"("Image In"=w500, "error in"=w498) -> ("Image Out"=w501:T8, "Calibrated Matches (Pattern Matching 1)"=w497:T3[], "error out"=w499:errorcluster)  [unwired: 22 in, 1 out]
              n139 = Index Array(array=w497) -> (element=w496:T3)  [unwired: 1 in]
              n140 = Unbundle By Name(w496) -> ("Position"=w492:cluster{"x":sgl, "y":sgl}, "Scale"=w495:sgl, "Score"=w493:sgl)
              n141 = Cluster To Array(cluster=w492) -> (array=w491:sgl[])
              n142 = Greater Than 0?(x=w495) -> (x > 0?=w494:bool)
            }
            frame Disabled {
              n143 = call "IMAQ Find Circles"("Max Radius"=sgl 1000.0, "error in (no error)"=w515, "Min Radius"=sgl 450.0, "Image Dst"=w504, "Image Src"=w504) -> ("error out"=w516:errorcluster, "Circles Data"=w513:T17, "Nb Circles"=w514:i32, "Image Dst Out"=w503:T8)  [unwired: 3 in]
              n144 = Index Array(array=w513) -> (element=w523:T18)  [unwired: 1 in]
              n145 = Unbundle By Name(w523) -> ("Pos. X"=w512:i32, "Pos. Y"=w511:i32, "Radius"=w507:i32)
              n146 = Multiply(x=w507, y=0.0004337631887456038) -> (x*y=w505:dbl)
              n147 = Build Array(w512, w511) -> (w510:i32[])
              n148 = Greater Than 0?(x=w514) -> (x > 0?=w519:bool)
              n149 = Array To Cluster(array=w510) -> (cluster=w509:cluster{"[0]":i32, "[1]":i32})
              n150 = call "IMAQ Convert Pixel to Real World"("error in (no error)"=w516, "Pixel Coordinates"=w509, "Calibrated Image"=w503) -> ("error out"=w521:errorcluster, "Real World Coordinates"=w522:cluster{"X":sgl, "Y":sgl}, "Calibrated Image (duplicate)"=w502:T8)  [unwired: 3 in, 3 out]
              n151 = Cluster To Array(cluster=w522) -> (array=w520:sgl[])
              n152 = call <vilib>:"Clear Errors.vi"("error in (no error)"=w521) -> ("error out"=w508:errorcluster)  [unwired: 5 in, 1 out]
            }
          }
        }
        frame "HB CH2" {
          n153 = disable-structure shown="Enabled" {
            disable-tunnel: [w542 w547] -> w531
            disable-tunnel: w530 -> [w541 w546]
            disable-tunnel: [w540 w550] -> w529
            disable-tunnel: w528 -> [w539 w545]
            disable-tunnel: [w532 w548] -> w524
            disable-tunnel: [w537 _] -> _
            disable-tunnel: [w536 w549] -> w527
            disable-tunnel: [_ w544] -> w526
            disable-tunnel: [w534 w543] -> w525
            frame Enabled {
              n154 = call "Vision Assistant9"("Image In"=w541, "error in"=w539) -> ("Image Out"=w542:T8, "Calibrated Matches (Pattern Matching 1)"=w538:T19, "error out"=w540:errorcluster)  [unwired: 22 in, 1 out]
              n155 = Index Array(array=w538) -> (element=w537:T20)  [unwired: 1 in]
              n156 = Unbundle By Name(w537) -> ("Position"=w533:cluster{"x":sgl, "y":sgl}, "Scale"=w535:sgl, "Score"=w534:sgl)
              n157 = Cluster To Array(cluster=w533) -> (array=w532:sgl[])
              n158 = Greater Than 0?(x=w535) -> (x > 0?=w536:bool)
            }
            frame Disabled {
              n159 = call-poly "IMAQ Detect Shapes"("error in (no error)"=w545, "Match Options"=T11 {"Rotation"=FALSE, "Scale"=FALSE, "Occlusion"=TRUE, "Range Settings"=[]}, "Circle Descriptor"=cluster{"Min Radius":dbl, "Max Radius":dbl} {"Min Radius"=50.0, "Max Radius"=2000.0}, "Image"=w546) -> ("error out"=w556:errorcluster, "Number of Matches Returned"=w559:i32, "Circles"=w555:T15)  [unwired: 5 in]
              n160 = Index Array(array=w555) -> (element=w554:T16)  [unwired: 1 in]
              n161 = Greater Than 0?(x=w559) -> (x > 0?=w549:bool)
              n162 = Unbundle By Name(w554) -> ("Position"=w553:cluster{"X":sgl, "Y":sgl}, "Radius"=w544:dbl, "Score"=w543:dbl)
              n163 = call "IMAQ Convert Pixel to Real World"("error in (no error)"=w556, "Pixel Coordinates"=w553, "Calibrated Image"=w546) -> ("error out"=w551:errorcluster, "Real World Coordinates"=w552:cluster{"X":sgl, "Y":sgl}, "Calibrated Image (duplicate)"=w547:T8)  [unwired: 3 in, 3 out]
              n164 = Cluster To Array(cluster=w552) -> (array=w548:sgl[])
              n165 = call <vilib>:"Clear Errors.vi"("error in (no error)"=w551) -> ("error out"=w550:errorcluster)  [unwired: 5 in, 1 out]
            }
          }
        }
        frame "Hexaboard Circle" {
          n166 = call "Vision Assistant2"("Image In"=w571, "error in"=w569) -> ("Image Out"=w572:T8, "Fitted Circle (Find Circular Edge 1)"=w573:T14, "error out"=w562:errorcluster)  [unwired: 23 in]
          n167 = Unbundle By Name(w573) -> ("Center (Real-World)"=w561:cluster{"X":sgl, "Y":sgl}, "Average Strength"=w570:dbl, "Radius (Real-World)"=w568:dbl)
          n168 = Cluster To Array(cluster=w561) -> (array=w560:sgl[])
          n169 = Greater?(x=w568, y=0.2) -> (0:w564:bool)
          n170 = Less?(x=w568, y=0.24) -> (x < y?=w565:bool)
          n171 = And(x=w564, y=w565) -> (x .and. y?=w563:bool)
        }
        frame "V3 Sensor Circle" {
          n172 = call "Vision Assistant4"("Image In"=w585, "error in"=w582) -> ("Image Out"=w586:T8, "Fitted Circle (Find Circular Edge 1)"=w587:T14, "error out"=w583:errorcluster)  [unwired: 23 in]
          n173 = Unbundle By Name(w587) -> ("Center (Real-World)"=w575:cluster{"X":sgl, "Y":sgl}, "Average Strength"=w584:dbl, "Radius (Real-World)"=w577:dbl)
          n174 = Cluster To Array(cluster=w575) -> (array=w574:sgl[])
          n175 = Greater?(x=w577, y=0.1) -> (0:w578:bool)
          n176 = Less?(x=w577, y=0.15) -> (x < y?=w579:bool)
          n177 = And(x=w578, y=w579) -> (x .and. y?=w576:bool)
        }
        frame "sensor CH1 check" {
          n178 = disable-structure shown="Enabled" {
            disable-tunnel: [w604 w606] -> w594
            disable-tunnel: w593 -> [w603 w606]
            disable-tunnel: [w602 w605] -> w592
            disable-tunnel: w591 -> [w601 w605]
            disable-tunnel: [w599 _] -> w590
            disable-tunnel: [w598 _] -> w589
            disable-tunnel: [w595 _] -> w588
            frame Disabled {
              n179 = call "Vision Assistant3"("Image In"=w603, "error in"=w601) -> ("Image Out"=w604:T8, "Calibrated Matches (Pattern Matching 1)"=w600:T3[], "error out"=w602:errorcluster)  [unwired: 22 in, 1 out]
              n180 = Index Array(array=w600) -> (element=w599:T3)  [unwired: 1 in]
              n181 = Unbundle By Name(w599) -> ("Position"=w596:cluster{"x":sgl, "y":sgl}, "Scale"=w597:sgl)
              n182 = Greater Than 0?(x=w597) -> (x > 0?=w598:bool)
              n183 = Cluster To Array(cluster=w596) -> (array=w595:sgl[])
            }
            frame Enabled {
            }
          }
        }
        frame "HB CH1 check " {
          n184 = disable-structure shown="Enabled" {
            disable-tunnel: [w623 w625] -> w613
            disable-tunnel: w612 -> [w622 w625]
            disable-tunnel: [w621 w624] -> w611
            disable-tunnel: w610 -> [w620 w624]
            disable-tunnel: [w618 _] -> w609
            disable-tunnel: [w617 _] -> w608
            disable-tunnel: [w614 _] -> w607
            frame Disabled {
              n185 = call "Vision Assistant11"("Image In"=w622, "error in"=w620) -> ("Image Out"=w623:T8, "Calibrated Matches (Pattern Matching 1)"=w619:T3[], "error out"=w621:errorcluster)  [unwired: 22 in, 1 out]
              n186 = Index Array(array=w619) -> (element=w618:T3)  [unwired: 1 in]
              n187 = Unbundle By Name(w618) -> ("Position"=w615:cluster{"x":sgl, "y":sgl}, "Scale"=w616:sgl)
              n188 = Cluster To Array(cluster=w615) -> (array=w614:sgl[])
              n189 = Greater Than 0?(x=w616) -> (x > 0?=w617:bool)
            }
            frame Enabled {
            }
          }
        }
      }
      "pattern matching" <- w34
      "Used Edges (Adv. Straight Edge 1)" <- w33
      n190 = disable-structure shown="Enabled" {
        disable-tunnel: w59 -> [w120 w134]
        disable-tunnel: [w123 w134] -> w58
        disable-tunnel: w55 -> [w119 w133]
        disable-tunnel: [w121 w133] -> w52
        frame Enabled {
          # "Adds crosshair to screen"
          n191 = call "IMAQ GetImageSize"("Image"=w120, "error in (no error)"=w119) -> ("Y Resolution"=w110:i32, "X Resolution"=w112:i32, "error out"=w118:errorcluster)  [unwired: 2 in]
          n192 = Decrement(x=w110) -> (x-1=w109:i32)
          n193 = Decrement(x=w112) -> (x-1=w111:i32)
          n194 = Max & Min(x=w111, y=w109) -> (max(x,y)=w113:i32)  [unwired: 1 out]
          n195 = Divide(x=w111, y=2.0) -> (x/y=w115:dbl)
          n196 = Subtract(x=w115, y=w113) -> (x-y=w124:dbl)
          n197 = Add(x=w115, y=w113) -> (x+y=w125:dbl)
          n198 = Divide(x=w109, y=2.0) -> (x/y=w114:dbl)
          n199 = Subtract(x=w114, y=w113) -> (x-y=w128:dbl)
          n200 = Add(x=w114, y=w113) -> (x+y=w129:dbl)
          n201 = Bundle(w124, w114) -> (w127:cluster{dbl, dbl})  [unwired: 1 in]
          n202 = Bundle(w125, w114) -> (w126:cluster{dbl, dbl})  [unwired: 1 in]
          n203 = call "IMAQ Overlay Line"("error in (no error)"=w118, "End Point"=w126, "Start Point"=w127, "Image"=w120) -> ("error out"=w122:errorcluster, "Image Out"=w132:T8)  [unwired: 6 in]
          n204 = Bundle(w115, w128) -> (w130:cluster{dbl, dbl})  [unwired: 1 in]
          n205 = Bundle(w115, w129) -> (w131:cluster{dbl, dbl})  [unwired: 1 in]
          n206 = call "IMAQ Overlay Line"("error in (no error)"=w122, "End Point"=w131, "Start Point"=w130, "Image"=w132) -> ("error out"=w121:errorcluster, "Image Out"=w123:T8)  [unwired: 6 in]
        }
        frame Disabled {
        }
      }
      n207 = disable-structure shown="Enabled" {
        disable-tunnel: w58 -> [w105 _]
        disable-tunnel: w52 -> [w104 w108]
        disable-tunnel: [w107 w108] -> w51
        disable-tunnel: [w106 _] -> w40
        frame Enabled {
          n208 = call "IMAQ Quantify 2"("error in (no error)"=w104, "Image"=w105) -> ("error out"=w107:errorcluster, "Global Report"=w106:T21)  [unwired: 7 in, 1 out]
        }
        frame Disabled {
        }
      }
      n209 = Bundle By Name(cluster="Image Indicators", "Average Strength"=w44, "Radius (Real-World)"=w43, "Match found?"=w42, "initial angle"=w41, "Global Report"=w40) -> (→"output cluster":T4)
    }
    frame Error {
    }
  }
  "error out" <- w11
  "Camera out" <- w10
  "Camera" <- w4
  "Image" <- w8
  "All Matches XY" <- w1
